vi "Analog Input (Host).vi"() -> ()   [LabVIEW 2011]
doc: "This VI will will initialize the FPGA VI and then continually read and calibrate single point values from 4 channels of an analog input module."
uses:
  <vilib>/rvi/interface/nirviReadWriteControl/nirviReadWriteControl.xnode
  <vilib>/rvi/interface/nirviCloseFPGA/nirviCloseFPGA.xnode
  <vilib>/rvi/interface/nirviOpenFPGA/nirviOpenFPGA.xnode
  FPGA Bitfiles/MAXCATProject_FPGATarget2_AnalogInput(FPGA_02AD9187.lvbitx
  Analog Input (FPGA).vi
  <vilib>/FPGAPlugInAG/cRIO-9074/niLvFpga_Open_cRIO-9074.vi
  <vilib>/rvi/interface/common/dynamic/niFpgaDynamicAddResources.vi
  NiFpgaLv.dll
  <vilib>/Utility/error.llb/Error Cluster From Error Code.vi
  <vilib>/rvi/interface/Simulation/niFpgaSimulationCallBeginRW.vi
  <vilib>/rvi/errors/niLvFpgaAdjustHostInterfaceError.vi
  <vilib>/FPGAPlugInAG/Dynamic/niLvFpga_Close_Dynamic.vi
panel:
  in  "Software Loop Time (ms)":u32=100
  out "Analog Input":T1(graph)={"cRIO-9211_TC_3[0]"=22.60995864868164, "cRIO-9211_TC_3[1]"=26.43000030517578, "cRIO-9211_TC_3[2]"=1414.2022705078125, "cRIO-9211_TC_3[3]"=1414.2022705078125}
  in  "stop":bool
  in  "AI Sample Rate (Hz)":dbl=10000.0
  # "For instructions, select  Help>>Show Context Help and hover over the icon."
  # "Resource Parameters"
  # "Timing Parameters"
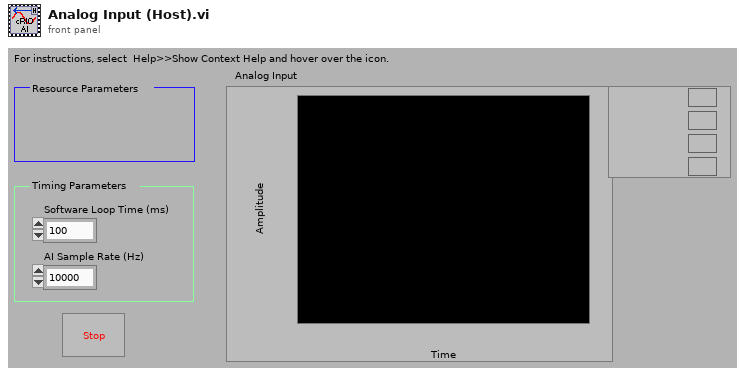
[diagram p1: front panel]
types:
  T1 = cluster{"cRIO-9211_TC_3[0]":dbl, "cRIO-9211_TC_3[1]":dbl, "cRIO-9211_TC_3[2]":dbl, "cRIO-9211_TC_3[3]":dbl}
  T2 = cluster{"Mod1/AI0":fxp<+/-,20,5>, "Mod1/AI1":fxp<+/-,20,5>, "Mod1/AI2":fxp<+/-,20,5>, "Mod1/AI3":fxp<+/-,20,5>}
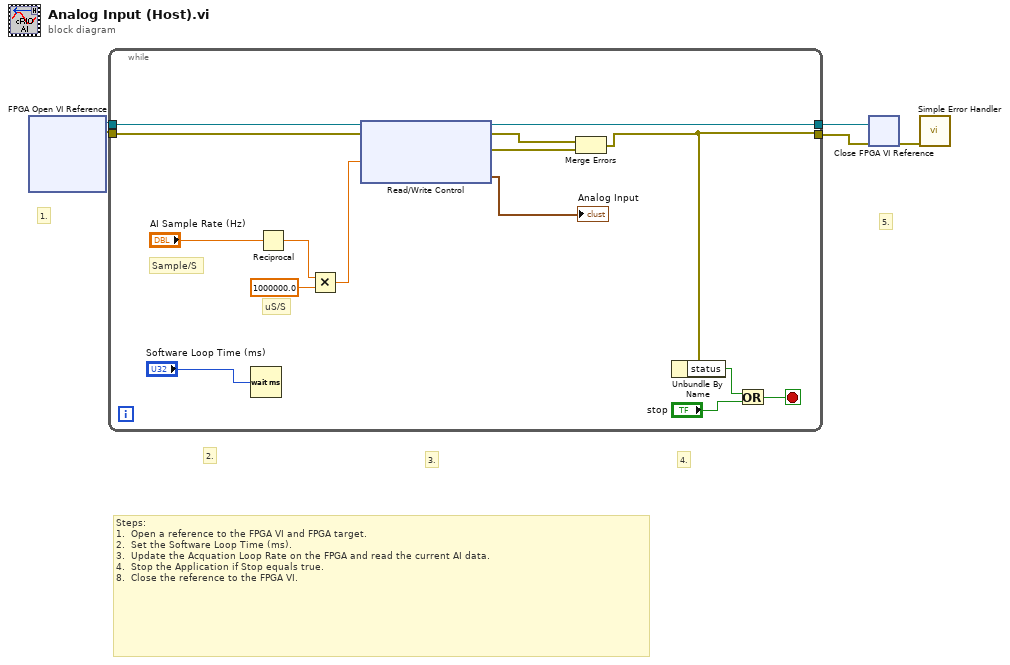
[diagram p0: block diagram]
diagram:
  # "5."
  # "3."
  # "4."
  # "2."
  # "1."
  # "Steps: \n1.  Open a reference to the FPGA VI and FPGA target.\n2.  Set the Software Loop Time (ms).\n3.  Update the Acquation Loop Rate on the FPGA and read the current AI data.\n4.  Stop the Application if Stop equals true. \n8.  Close the reference to the FPGA VI."
  n1 = xnode "FPGA Open VI Reference"() -> ("FPGA VI Reference Out"=w2:refnum<k20>, "error out"=w1:errorcluster)  [unwired: 2 in]
  n2 = while {
    tunnel: w2 -> [w11]
    tunnel: w1 -> [w10]
    tunnel: [w8] -> w5
    tunnel: [w9] -> w4
    stop <- w19 stop-if-true
    # "Sample/S"
    # "uS/S"
    n3 = Wait (ms)(milliseconds to wait="Software Loop Time (ms)") -> ()  [unwired: 1 out]
    n4 = Reciprocal(x="AI Sample Rate (Hz)") -> (1/x=w17:dbl)
    n5 = Multiply(x=w17, y=1000000.0) -> (x*y=w15:dbl)
    n6 = xnode "Read/Write Control"("FPGA VI Reference In"=w11, "error in"=w10, "AI Sample Rate(uSec)"=w15) -> ("FPGA VI Reference Out"=w8:refnum<k20>, "error out"=w14:errorcluster, "FPGA Error Out"=w13:errorcluster, "AI Data"=→"Analog Input":T2)
    n7 = Merge Errors(w14, w13) -> (w9:errorcluster)
    n8 = Unbundle By Name(w9) -> ("status"=w18:bool)
    n9 = Or(x=w18, y="stop") -> (x .or. y?=w19:bool)
  }
  n10 = xnode "Close FPGA VI Reference"("FPGA VI Reference In"=w5, "error in"=w4) -> ("error out"=w3:errorcluster)
  n11 = call <vilib>:"Simple Error Handler.vi"("error in (no error)"=w3) -> ()  [unwired: 1 in, 8 out]
